vi "Write Simulated.vi"(8 "error in (no error)":errorcluster, 10 "Simulated":bool, 11 "Controller in":refnum<class "Controller.lvclass">) -> (0 "error out":errorcluster, 3 "Controller out":refnum<class "Controller.lvclass">)   [LabVIEW 2019, in "Controller.lvlib" / "Controller.lvclass"]
uses:
  Controller.lvclass
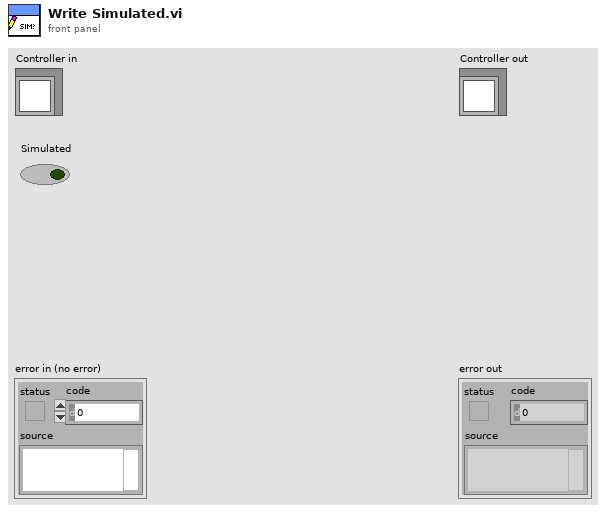
[diagram p1: front panel]
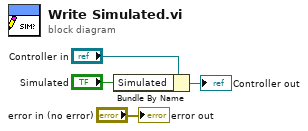
[diagram p0: block diagram]
diagram:
  n1 = Bundle By Name(cluster="Controller in", "Simulated"="Simulated") -> (→"Controller out":refnum<class "Controller.lvclass">)
  "error out" <- "error in (no error)"
